vi "Increment PC.vi"(8 "error in (no error)":errorcluster, 11 "gScript Interpreter in":refnum<class "gScript Interpreter.lvclass">) -> (0 "error out":errorcluster, 2 "Finished":bool, 3 "gScript Interpreter out":refnum<class "gScript Interpreter.lvclass">)   [LabVIEW 2017, in "gScript Interpreter.lvclass"]
uses:
  gScript Interpreter.lvclass
  gScript Interpreter.lvclass/gScript Interpreter.ctl
  Type Definitions/Command.ctl
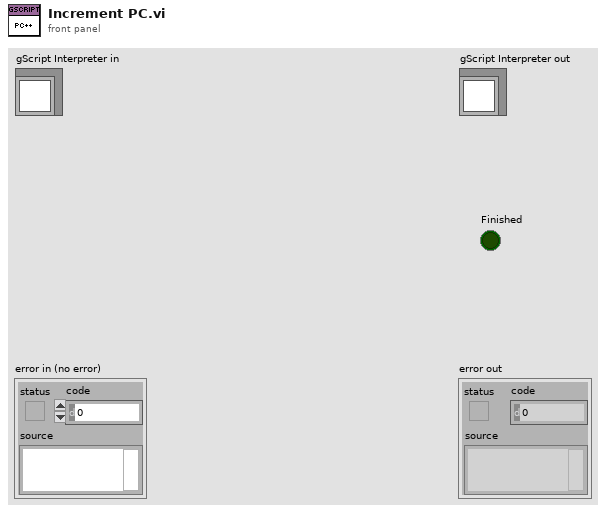
[diagram p1: front panel]
types:
  T1 = typedef "Command.ctl" = enum16{"", "PASS", "COPY", "PRINT", "GOTO", "GOTOIF", "GOTOIFN", "ADD", "SUB", "INC", "DEC", "HOME", "MOVEREL", "MOVENAME", "MOVETO", "GETPOS", "ROTATE", "GETROT", "SETVAC", "GETVAC", "JOYSTICK", "LOADTOOL", "UNLOADTOOL", "POTLINE", "POTDOT", "AUTOFOCUS", "FINDFID", "FIT", "WAIT", "MPGON", "MPGOFF", "PAUSE", "SNAPSHOT", "SETLOG", "CLEARLOG", "VIDEO", "TRANSFORMG2L", "TRANSFORML2G", "CHOICEPOPUP", "SETLIGHT", "CALL", "END", "DUMPSTATE", "FLEXREAD", "FLEXWRITE", "SURVEY", "LOADCONFIG", "SETERRORMODE", "COMPOSE", "INVERT", "EULER2QUAT", "QUAT2EULER", "MUL", "ROTATETO", "VERSION", "SIN", "COS", "TAN", "ATAN2", "ABS", "POW", "ACKFAULT", "MOVESAFE", "LOADSTAMP", "APPLYSTAMP", "UNLOADSTAMP", "LOADWEIGHT", "APPLYWEIGHT", "UNLOADWEIGHT", "RETURN", "GETFLOATPOPUP", "GETINTPOPUP", "GETVECPOPUP", "CLEARVARS"}
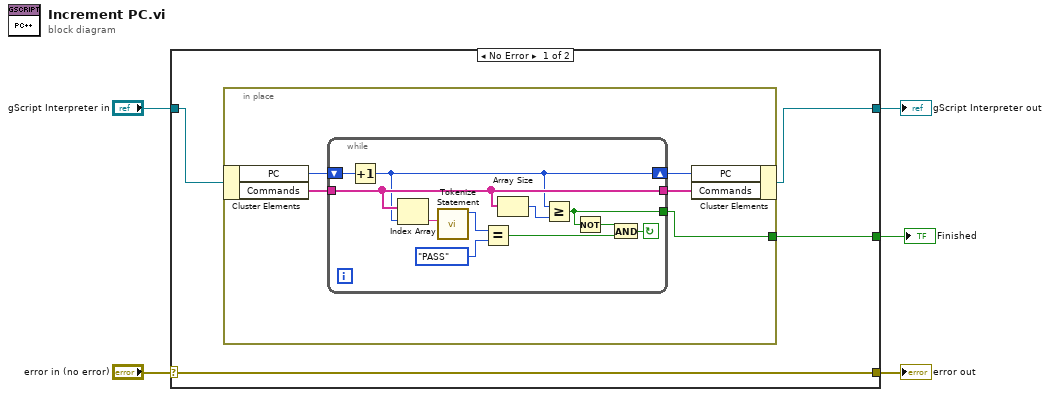
[diagram p0: block diagram]
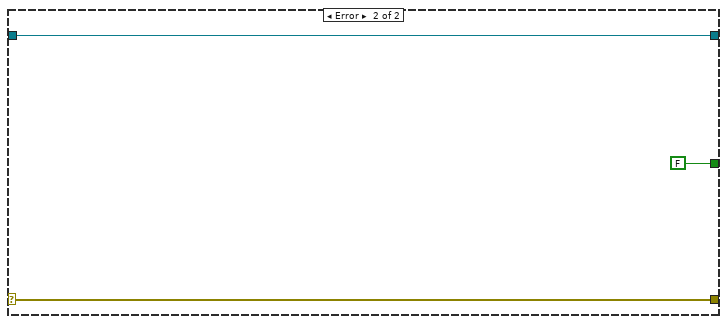
[diagram p2: hidden frame]
diagram:
  n1 = case shown="No Error" "error in (no error)" {
    selector: "error in (no error)" -> [w9 w28]
    tunnel: [w9 w28] -> w4
    tunnel: [w7 w27] -> w2
    tunnel: "gScript Interpreter in" -> [w8 w27]
    tunnel: [w6 FALSE] -> w1
    frame No Error {
      n2 = in-place {
        in-place-border: [w10] -> w6
        n3 = in-place-cluster #1(w8) -> ("PC"=w13:i32, "Commands"=w14:string[])
        n4 = while {
          tunnel: w14 -> [w20]
          shift-right: [w19] -> w12
          shift-left: w13 -> [w24]
          tunnel: [w20] -> w11
          tunnel: [w16] -> w10
          stop <- w17 continue-if-true
          n5 = Increment(x=w24) -> (x+1=w19:i32)
          n6 = Index Array(array=w20, index=w19) -> (element=w25:string)
          n7 = call "Tokenize Statement.vi"("Command"=w25) -> ("Command"=w23:T1)  [unwired: 6 in, 4 out]
          n8 = Equal?(x=w23, y=Command."PASS") -> (x = y?=w18:bool)
          n9 = Array Size(array=w20) -> (size(s)=w21:i32)
          n10 = Greater Or Equal?(x=w19, y=w21) -> (x >= y?=w16:bool)
          n11 = Not(x=w16) -> (.not. x?=w15:bool)
          n12 = And(x=w15, y=w18) -> (x .and. y?=w17:bool)
        }
        n13 = in-place-cluster #1("PC"=w12, "Commands"=w11) -> (w7:refnum<class "gScript Interpreter.lvclass">)
      }
    }
    frame Error {
    }
  }
  "error out" <- w4
  "gScript Interpreter out" <- w2
  "Finished" <- w1
